vi "FW Set Speed.vi"(0 "Notifier Name In":string, 2 "Wait for Finish":bool=TRUE, 7 "Speed":dbl, 11 "Error In":errorcluster) -> (4 "Notifier Name Out":string, 15 "Error Out":errorcluster)   [LabVIEW 2020]
uses:
  FW Type Defs/FW Notifier Type.ctl
  FW Type Defs/FW Actions.ctl
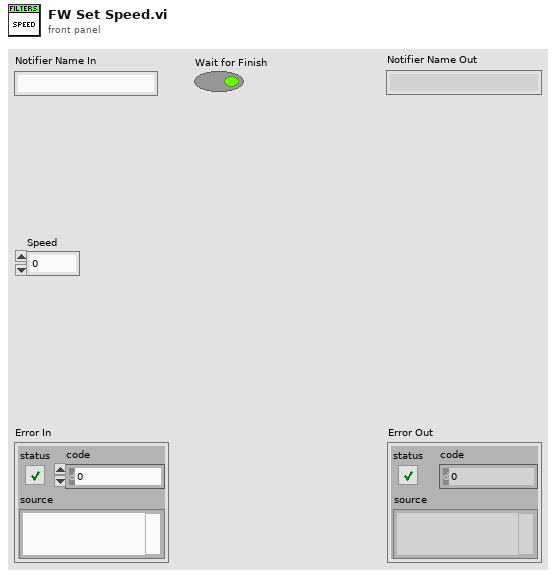
[diagram p1: front panel]
types:
  T1 = typedef "FW Notifier Type.ctl" = cluster{"Actions":T2, "Set Position":u8, "Actual Position":u8, "Speed":dbl, "Num Positions":u8, "Received":bool}
  T2 = typedef "FW Actions.ctl" = enum16{"Set Position", "Get Position", "Get Num Positions", "Set Speed", "Confirm Pos", "Quit"}
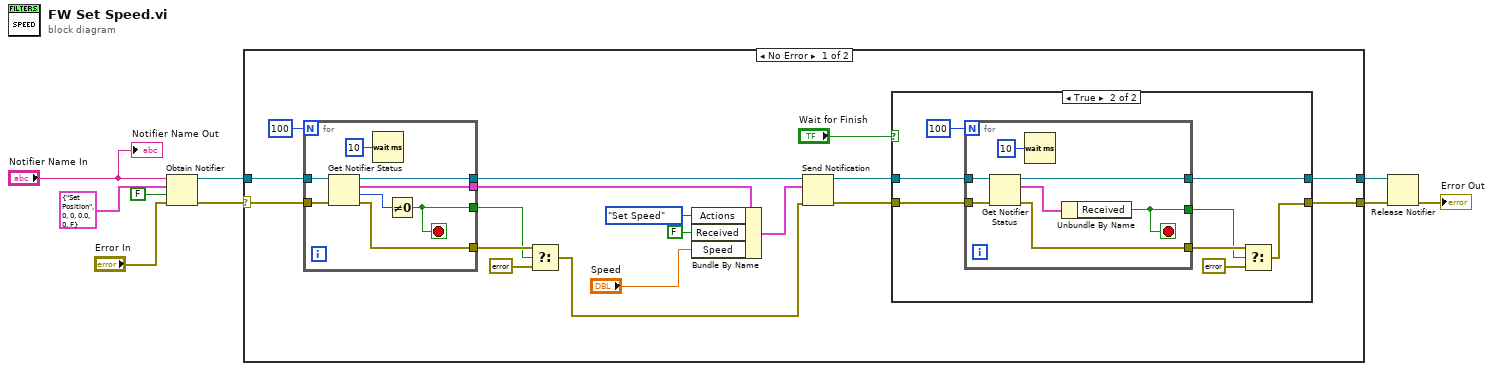
[diagram p0: block diagram]
diagram:
  n1 = Obtain Notifier(name (unnamed)="Notifier Name In", notification data type=T1 {"Actions"=enum."Set Position", "Set Position"=0, "Actual Position"=0, "Speed"=0.0, "Num Positions"=0, "Received"=FALSE} ("FW102C Note Type"), create if not found? (T)=FALSE, error in (no error)="Error In") -> (notifier out=w6:refnum<notifier>, error out=w7:errorcluster)  [unwired: 1 out]
  n2 = case shown="No Error" w7 {
    selector: w7 -> [w25 w54]
    tunnel: w6 -> [w27 w53]
    tunnel: [w19 w54] -> w3
    tunnel: [w20 w53] -> w4
    frame No Error {
      n3 = for {
        N: 100 -> [_]
        tunnel: w27 -> [w52]
        tunnel: [w50] -> w16
        tunnel: [w48] -> w24
        tunnel: w25 -> [w47]
        tunnel: [w46] -> w17
        tunnel: [w45] -> w12
        stop <- w50 stop-if-true
        n4 = Get Notifier Status(notifier=w52, error in (no error)=w47) -> (notifier out=w48:refnum<notifier>, current notification=w45:T1, # waiting=w51:i32, error out=w46:errorcluster)  [unwired: 1 out]
        n5 = Wait (ms)(milliseconds to wait=u32 10) -> ()  [unwired: 1 out]
        n6 = Not Equal To 0?(x=w51) -> (x != 0?=w50:bool)
      }
      n7 = Select(t=w17, s=w16, f=errorcluster {"status"=TRUE, "code"=0, "source"="Filter wheel busy. Timeout error."}) -> (s? t:f=w11:errorcluster)
      n8 = Bundle By Name(cluster=w12, "Actions"=FW_Actions."Set Speed", "Received"=FALSE, "Speed"="Speed") -> (w23:T1)
      n9 = Send Notification(notification=w23, notifier=w24, error in (no error)=w11) -> (notifier out=w21:refnum<notifier>, error out=w22:errorcluster)
      n10 = case shown="True" "Wait for Finish" {
        tunnel: w22 -> [w28 w37]
        tunnel: w21 -> [w29 w36]
        tunnel: [w29 w35] -> w20
        tunnel: [w28 w34] -> w19
        frame False {
        }
        frame True {
          n11 = for {
            N: 100 -> [_]
            tunnel: w36 -> [w44]
            tunnel: [w42] -> w35
            tunnel: w37 -> [w41]
            tunnel: [w40] -> w32
            tunnel: [w38] -> w31
            stop <- w38 stop-if-true
            n12 = Get Notifier Status(notifier=w44, error in (no error)=w41) -> (notifier out=w42:refnum<notifier>, current notification=w39:T1, error out=w40:errorcluster)  [unwired: 2 out]
            n13 = Wait (ms)(milliseconds to wait=u32 10) -> ()  [unwired: 1 out]
            n14 = Unbundle By Name(w39) -> ("Received"=w38:bool)
          }
          n15 = Select(t=w32, s=w31, f=errorcluster {"status"=TRUE, "code"=0, "source"="Filter Wheel Error: Action didn't complete."}) -> (s? t:f=w34:errorcluster)
        }
      }
    }
    frame Error {
    }
  }
  n16 = Release Notifier(notifier=w4, error in (no error)=w3) -> (error out=→"Error Out":errorcluster)  [unwired: 1 in, 2 out]
  "Notifier Name Out" <- "Notifier Name In"
